vi "Interruptible Timer Monitor.vi"(5 "Max":dbl format="%#_13g", 7 "Min":dbl format="%#_13g", 8 "error in (no error)":errorcluster, 10 "Update UI?":bool, 11 "Wait (s)":i32) -> (0 "error out":errorcluster, 1 "In Range?":bool, 2 "Leak Rate":dbl, 3 "Aborted?":bool, 4 "NI-DAQ Pressure":dbl)   [LabVIEW 2015]
uses:
  User Interface/UI Handler/UI Handler.lvclass
  Common/State Machine/State Machine.lvlib
  Common/Buffers/Circular Buffer/Circular Buffer.lvclass
  <vilib>/Analysis/NI_AALPro.lvlib
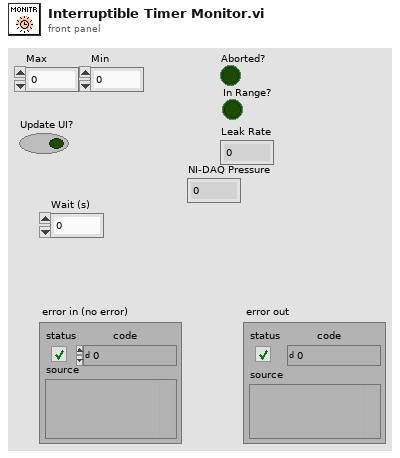
[diagram p1: front panel]
types:
  T1 = cluster{"result string":string, "current time":timestamp}
  T2 = typedef "Circular Buffer.lvclass/Session Handle.ctl" = refnum<data-value>
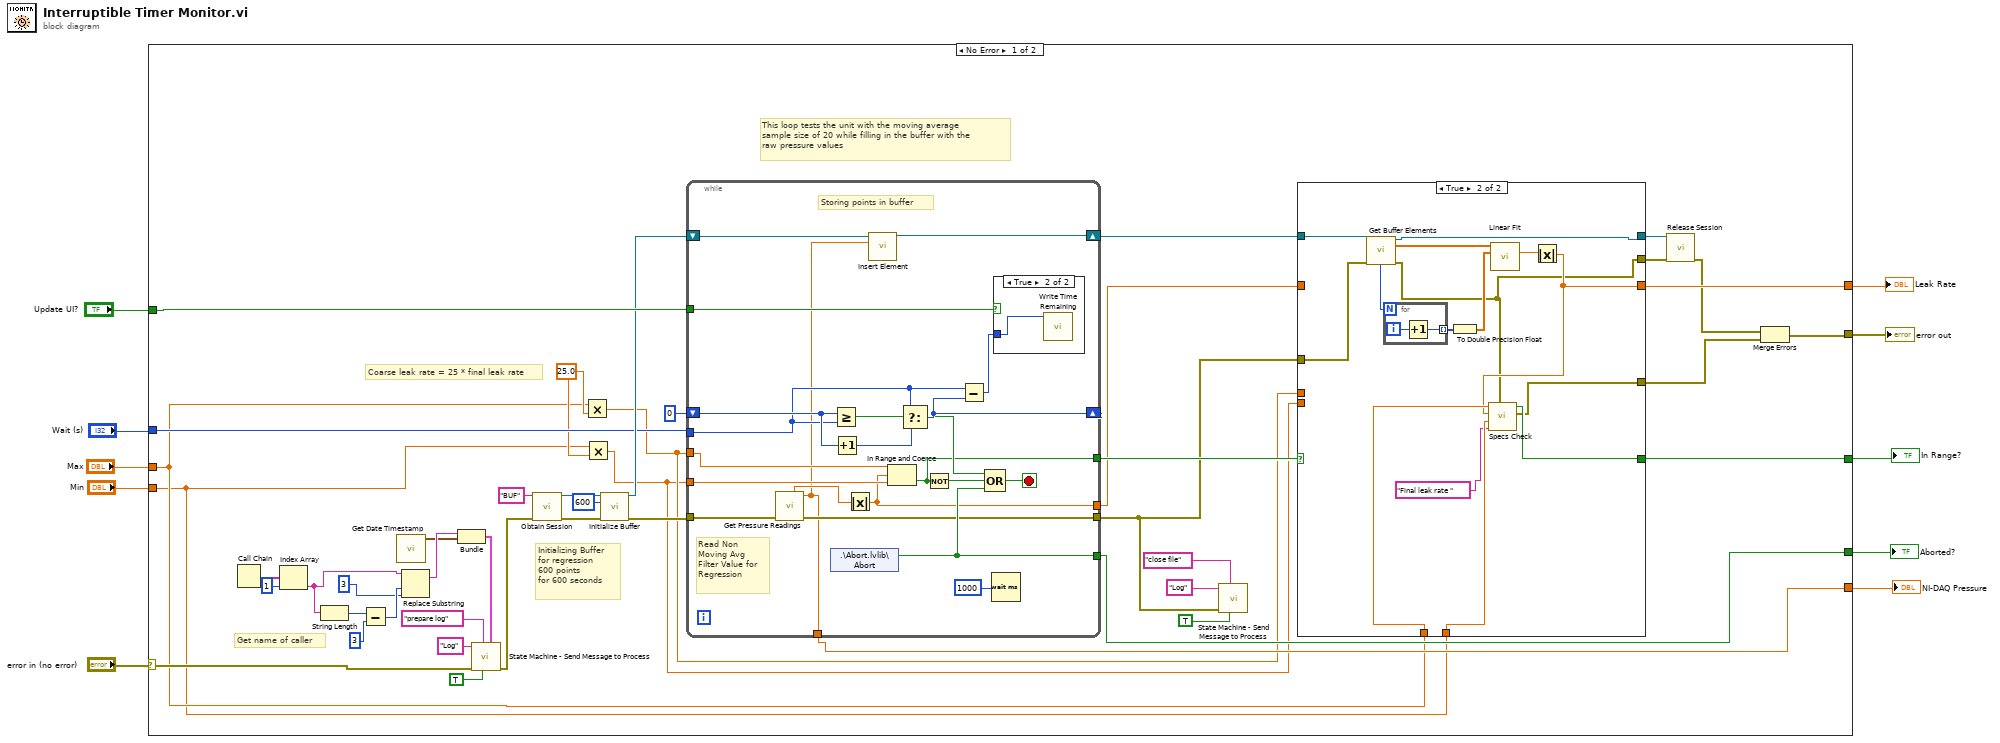
[diagram p0: block diagram]
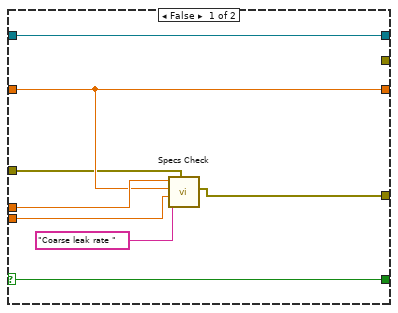
[diagram p2: hidden frame]
diagram:
  n1 = case shown="No Error" "error in (no error)" {
    selector: "error in (no error)" -> [w41 _]
    tunnel: "Update UI?" -> [w54 _]
    tunnel: "Max" -> [w19 _]
    tunnel: "Min" -> [w18 _]
    tunnel: "Wait (s)" -> [w29 _]
    tunnel: [w11 _] -> w5
    tunnel: [w25 _] -> w4
    tunnel: [w24 _] -> w3
    tunnel: [w23 _] -> w2
    tunnel: [w22 _] -> w1
    frame No Error {
      w20 = 25.0 ("y")
      # "Coarse leak rate = 25 * final leak rate"
      # "This loop tests the unit with the moving average\nsample size of 20 while filling in the buffer with the \nraw pressure values"
      # "Initializing Buffer\nfor regression\n600 points\nfor 600 seconds"
      # "Get name of caller"
      n2 = Call Chain() -> (call chain=w48:string[])
      n3 = Index Array(array=w48, index=1) -> (element=w44:string)
      n4 = String Length(string=w44) -> (length=w51:i32)
      n5 = Subtract(x=w51, y=3) -> (x-y=w53:i32)
      n6 = call "Get Date Timestamp.vi"() -> ("current time"=w37:timestamp)  [unwired: 10 in, 1 out]
      n7 = Replace Substring(2:3 ("length (len. of substring)"), 3:w53, 5:w44) -> (1:w43:string)  [unwired: 1 in, 1 out]
      n8 = Bundle("result string"=w43, "current time"=w37) -> (w42:T1)  [unwired: 1 in]
      n9 = call "State Machine - Send Message to Process.vi"("Data"=w42, "Front?"=TRUE, "State"="prepare log", "error in (no error)"=w41, "Process Name"="Log") -> ("error out"=w35:errorcluster)  [unwired: 6 in]
      n10 = call "Obtain Session.vi"("Session  Name ()"="BUF", "error in (no error)"=w35) -> ("Session Handle"=w33:T2, "error out"=w34:errorcluster)  [unwired: 12 in]
      n11 = Multiply(x=w19, y=w20) -> (x*y=w17:dbl)
      n12 = Multiply(x=w18, y=w20) -> (x*y=w16:dbl)
      n13 = call "Initialize Buffer.vi"("Session Handle in"=w33, "Size"=u16 600, "error in (no error)"=w34) -> ("Session Handle out"=w30:T2, "error out"=w31:errorcluster)  [unwired: 11 in]
      n14 = while {
        tunnel: w29 -> [w98]
        shift-right: [w99] -> _
        shift-left: 0 -> [w101]
        tunnel: [w93] -> w24
        tunnel: w54 -> [w96]
        tunnel: w16 -> [w94]
        tunnel: w31 -> [w87]
        tunnel: [w91] -> w26
        tunnel: [w84] -> w28
        shift-right: [w86] -> w27
        shift-left: w30 -> [w88]
        tunnel: [w81] -> w23
        tunnel: [w83] -> w21
        tunnel: w17 -> [w82]
        stop <- w85 stop-if-true
        # "Storing points in buffer"
        # "Read Non\nMoving Avg\nFilter Value for\nRegression"
        n15 = call "Get Pressure Readings.vi"("error in (no error)"=w87) -> ("error out"=w91:errorcluster, "NI-DAQ Pressure"=w81:dbl, "Instantaneous"=w89:dbl)  [unwired: 7 in, 1 out]
        n16 = shared-variable ".\\Abort.lvlib\\Abort"() -> (w93:bool)  [unwired: 1 in, 1 out]
        n17 = Greater Or Equal?(x=w101, y=w98) -> (x >= y?=w95:bool)
        n18 = Increment(x=w101) -> (x+1=w100:i32)
        n19 = Absolute Value(x=w89) -> (abs(x)=w83:dbl)
        n20 = call "Insert Element.vi"("Session Handle in"=w88, "Value"=w81) -> ("Session Handle out"=w86:T2)  [unwired: 12 in, 1 out]
        n21 = In Range and Coerce(upper limit=w82, x=w83, lower limit=w94) -> (In Range?=w84:bool)  [unwired: 1 out]
        n22 = Select(t=w98, s=w95, f=w100) -> (s? t:f=w99:i32)
        n23 = Not(x=w84) -> (.not. x?=w92:bool)
        n24 = Subtract(x=w98, y=w99) -> (x-y=w97:i32)
        n25 = Compound Arithmetic op=OR(w95, w92, w93) -> (w85:bool)
        n26 = Wait (ms)(milliseconds to wait=u32 1000) -> ()  [unwired: 1 out]
        n27 = case shown="True" w96 {
          tunnel: w97 -> [_ w102]
          frame False {
          }
          frame True {
            n28 = call "Write Time Remaining.vi"("Value"=w102) -> ()  [unwired: 10 in, 1 out]
          }
        }
      }
      n29 = call "State Machine - Send Message to Process.vi"("Front?"=TRUE, "State"="close file", "error in (no error)"=w26, "Process Name"="Log") -> ()  [unwired: 7 in, 1 out]
      n30 = case shown="True" w28 {
        selector: w28 -> [w63 _]
        tunnel: w27 -> [w62 w73]
        tunnel: w19 -> [_ w70]
        tunnel: w18 -> [_ w68]
        tunnel: w26 -> [w56 w72]
        tunnel: [w63 w67] -> w25
        tunnel: [w59 w69] -> w22
        tunnel: w21 -> [w59 _]
        tunnel: w17 -> [w61 _]
        tunnel: w16 -> [w60 _]
        tunnel: [w62 w71] -> w15
        tunnel: [w57 w65] -> w13
        tunnel: [_ w64] -> w14
        frame False {
          n31 = call "Specs Check.vi"("error in"=w56, "parameter"="Coarse leak rate " ("initial string"), "lower limit"=w60, "x"=w59, "upper limit"=w61) -> ("error out"=w57:errorcluster)  [unwired: 5 in, 1 out]
        }
        frame True {
          n32 = call "Get Buffer Elements.vi"("Session Handle in"=w73, "error in (no error)"=w72) -> ("Session Handle out"=w71:T2, "Values"=w74:dbl[], "Counter"=w76:u16, "error out"=w64:errorcluster)  [unwired: 10 in]
          n33 = for {
            N: w76 -> [_]
            tunnel: [w79] -> w75 mode=indexing
            i -> [w80]
            n34 = Increment(x=w80) -> (x+1=w79:i32)
          }
          n35 = To Double Precision Float(number=w75) -> (double precision float=w77:dbl[])
          n36 = call <vilib>:"Linear Fit.vi"("Y"=w74, "X"=w77) -> ("slope"=w78:dbl)  [unwired: 9 in, 4 out]
          n37 = Absolute Value(x=w78) -> (abs(x)=w69:dbl)
          n38 = call "Specs Check.vi"("error in"=w64, "parameter"="Final leak rate " ("initial string"), "lower limit"=w68, "x"=w69, "upper limit"=w70) -> ("error out"=w65:errorcluster, "In Range?"=w67:bool)  [unwired: 5 in]
        }
      }
      n39 = call "Release Session.vi"("Session Handle"=w15, "error in (no error)"=w14) -> ("error out"=w12:errorcluster)  [unwired: 13 in]
      n40 = Merge Errors(w12, w13) -> (w11:errorcluster)
    }
    frame Error {
    }
  }
  "error out" <- w5
  "In Range?" <- w4
  "Aborted?" <- w3
  "NI-DAQ Pressure" <- w2
  "Leak Rate" <- w1
